vi "AlliGator Save Calibration Phasor.vi"(8 "Error In":errorcluster, 11 "Calibration Phasor":T1) -> (0 "error out":errorcluster, 1 "Message":string, 3 "XML File Path":path)   [LabVIEW 2021, in "AlliGator Phasor Calibration.lvlib"]
doc: "Saves the <B>Phasor Calibration</B>."
uses:
  Phasor/Calibration Phasor (m, phi).ctl
  AlliGator Phasor Calibration.lvlib
  Files/Files.lvlib
  Phasor/Phasor.lvlib
panel:
  # "see the AlliGator License on the block diagram (Ctrl+E or Window:Show Block Diagram)"
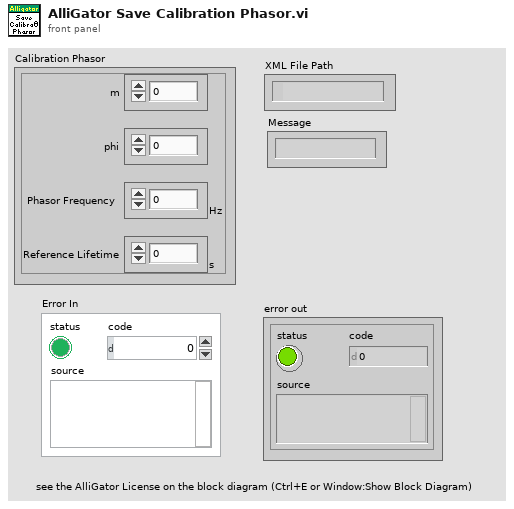
[diagram p1: front panel]
types:
  T1 = typedef "Phasor.lvlib/Calibration Phasor (m, phi).ctl" = cluster{"m":dbl, "phi":dbl, "Phasor Frequency":dbl[unit], "Reference Lifetime":dbl[unit]}
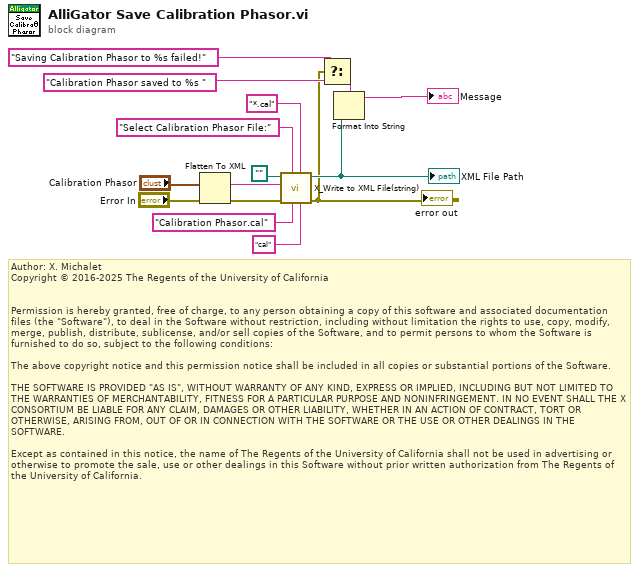
[diagram p0: block diagram]
diagram:
  # "Author: X. Michalet\nCopyright © 2016-2025 The Regents of the University of California\n \n\nPermission is hereby granted, free of charge, to any person obtaining a copy of this software and associated documentation files (the \"Software\"), to deal in the Software without restriction, including without limitation the rights to use, copy, modify, merge, publish, distribute, sublicense, and/or sell copies of the Software, and to permit persons to whom the Software is furnished to do so, subject to the following conditions:\n\nThe above copyright notice and this permission notice shall be included in all copies or substantial portions of the Software.\n\nTHE SOFTWARE IS PROVIDED \"AS IS\", WITHOUT WARRANTY OF ANY KIND, EXPRESS OR IMPLIED, INCLUDING BUT NOT LIMITED TO THE WARRANTIES OF MERCHANTABILITY, FITNESS FOR A PARTICULAR PURPOSE AND NONINFRINGEMENT. IN NO EVENT SHALL THE X CONSORTIUM BE LIABLE FOR ANY CLAIM, DAMAGES OR OTHER LIABILITY, WHETHER IN AN ACTION OF CONTRACT, TORT OR OTHERWISE, ARISING FROM, OUT OF OR IN CONNECTION WITH THE SOFTWARE OR THE USE OR OTHER DEALINGS IN THE SOFTWARE.\n\nExcept as contained in this notice, the name of The Regents of the University of California shall not be used in advertising or otherwise to promote the sale, use or other dealings in this Software without prior written authorization from The Regents of the University of California."
  n1 = Flatten To XML(6:"Calibration Phasor") -> (2:w13:string)
  n2 = call "X_Write to XML File(string).vi"("File Extension (xml)"="cal", "Pattern (*.xml;*.XML)"="*.cal", "default name"="Calibration Phasor.cal", "Prompt"="Select Calibration Phasor File:", "error in (no error)"="Error In", "XML Input"=w13, "XML File Start Path"=path "") -> ("error out"=w3:errorcluster, "XML File Path"=w12:path)  [unwired: 1 in, 2 out]
  "XML File Path" <- w12
  "error out" <- w3
  n3 = Select(t="Saving Calibration Phasor to %s failed!" ("format string"), s=w3, f="Calibration Phasor saved to %s " ("format string")) -> (s? t:f=w11:string)
  n4 = Format Into String(format string=w11, w12) -> (resulting string=→"Message":string)  [unwired: 2 in, 1 out]
